vi "DAQmxMappingLookup.vi"() -> ()   [LabVIEW 2024, in "Shared Steps.lvlib"]
uses:
  Shared Steps.lvlib
  <resource>/objmgr/daqmx.rc
panel:
  out "Mappings":T1(array[cluster])
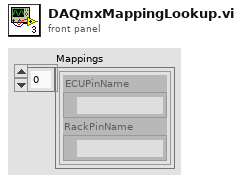
[diagram p1: front panel]
types:
  T1 = cluster{"ECUPinName":refnum<k21>, "RackPinName":tag}[]
  T2 = cluster{"ECUPinName":refnum<k21>, "RackPinName":tag}
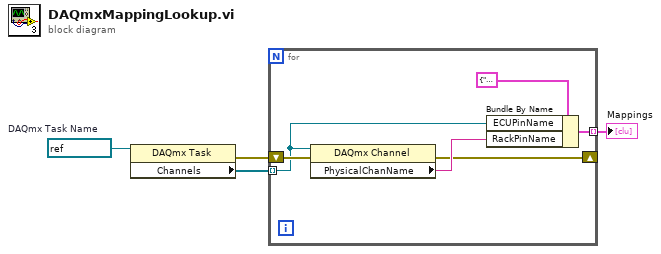
[diagram p0: block diagram]
diagram:
  w4 = refnum<k21> "RackAI"  # DAQmx Task Name
  n1 = property class="DAQmx Task"(reference=w4) -> (error out=w2:errorcluster, "Channels"=w3:refnum<k21>[])  [unwired: 1 in, 1 out]
  n2 = for {
    tunnel: w3 -> [w9] mode=indexing
    tunnel: [w7] -> w1 mode=indexing
    shift-right: [w6] -> _
    shift-left: w2 -> [w10]
    n3 = property class="DAQmx Channel"(reference=w9, error in=w10) -> (error out=w6:errorcluster, "PhysicalChanName"=w8:tag)  [unwired: 1 out]
    n4 = Bundle By Name(cluster=T2 {"ECUPinName"="", "RackPinName"=""}, "ECUPinName"=w9, "RackPinName"=w8) -> (w7:T2)
  }
  "Mappings" <- w1
